vi "Insert Into Subpanel.vi"(8 "error in (no error)":errorcluster, 9 "Insertion Request Time":timestamp, 10 "Viewable":refnum<class "IViewable.lvclass">, 11 "Protected Subpanel":T1) -> (0 "error out":errorcluster, 1 "Inserted?":bool, 2 "Viewable Out":refnum<class "IViewable.lvclass">, 3 "Protected Subpanel":T1)   [LabVIEW 2020, in "MVA Framework.lvlib" / "IViewable.lvlib" / "ProtectedSubpanel.lvclass"]
doc: "插入子面板"
uses:
  ProtectedSubpanel.lvclass
  Protected Subpanel Reference.ctl
  IViewable/IViewable.lvclass
  IViewable/IViewable.lvclass/IViewable.ctl
  ProtectedSubpanel.lvclass/ProtectedSubpanel.ctl
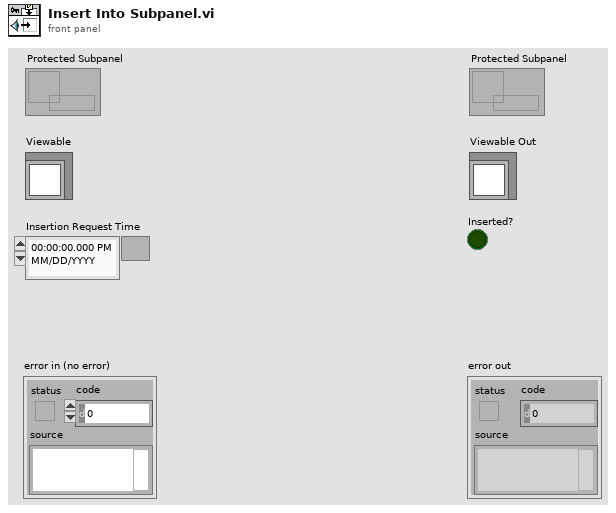
[diagram p1: front panel]
types:
  T1 = typedef "MVA Framework.lvlib/IViewable.lvlib/ProtectedSubpanel.lvclass/Protected Subpanel Reference.ctl" = refnum<data-value>
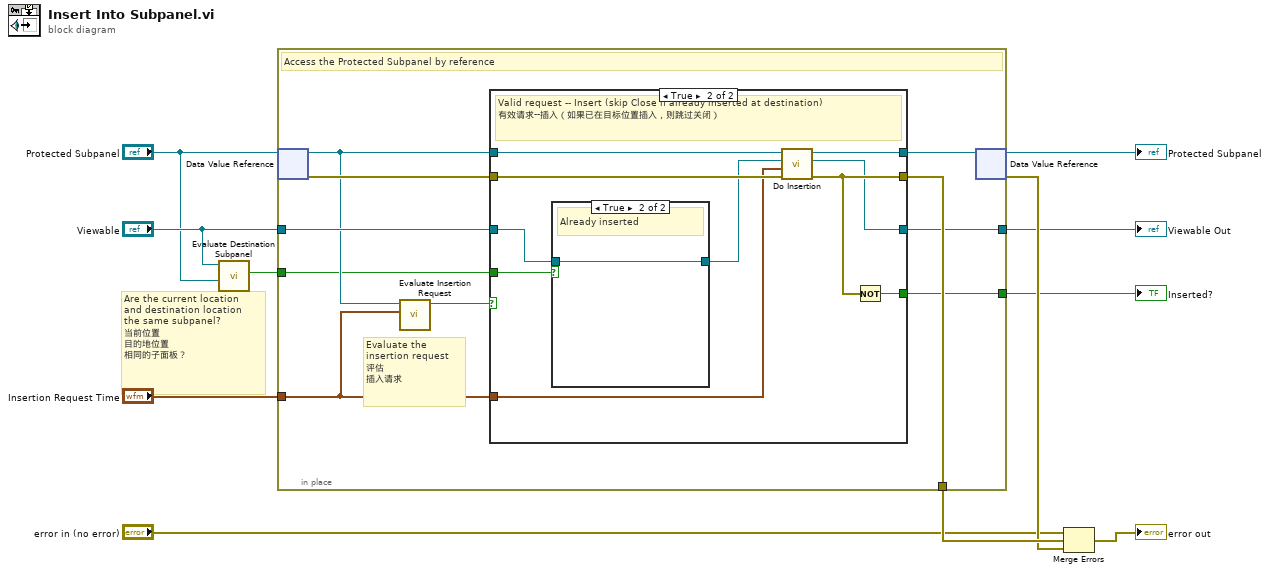
[diagram p0: block diagram]
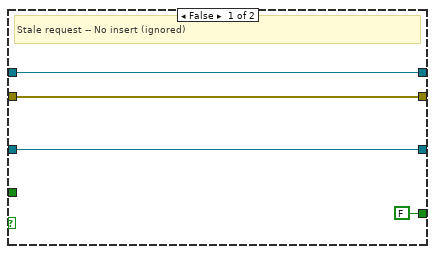
[diagram p2: hidden frame]
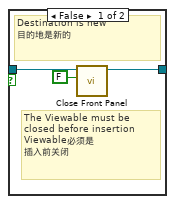
[diagram p3: hidden frame]
diagram:
  # "Are the current location\nand destination location\nthe same subpanel?\n当前位置\n目的地位置\n相同的子面板？"
  n1 = call "Evaluate Destination Subpanel.vi"("Destination Subpanel"="Protected Subpanel", "Viewable in"="Viewable") -> ("Already Inserted?"=w2:bool)  [unwired: 9 in]
  n2 = in-place {
    in-place-border: "Viewable" -> [w15]
    in-place-border: "Insertion Request Time" -> [w17]
    in-place-border: [w18] -> w8
    in-place-border: [w16] -> w6
    in-place-border: [w13] -> w5
    in-place-border: w2 -> [w12]
    # "Evaluate the\ninsertion request\n评估\n插入请求"
    # "Access the Protected Subpanel by reference"
    n3 = in-place-dvr #1("Protected Subpanel") -> (w14:refnum<class "ProtectedSubpanel.lvclass">, w19:errorcluster)
    n4 = call "Evaluate Insertion Request.vi"("Insertion Request Time"=w17, "ProtectedSubpanel"=w14) -> ("Perform Insertion?"=w20:bool)  [unwired: 9 in]
    n5 = case shown="True" w20 {
      tunnel: [w25 w35] -> w21
      tunnel: w14 -> [w25 w34]
      tunnel: w19 -> [w24 w33]
      tunnel: [w24 w32] -> w18
      tunnel: w17 -> [_ w30]
      tunnel: [FALSE w31] -> w16
      tunnel: w15 -> [w22 w28]
      tunnel: [w22 w29] -> w13
      tunnel: w12 -> [_ w26]
      frame False {
        # "Stale request -- No insert (ignored)"
      }
      frame True {
        # "Valid request -- Insert (skip Close if already inserted at destination)\n有效请求--插入（如果已在目标位置插入，则跳过关闭）"
        n6 = case shown="True" w26 {
          tunnel: w28 -> [w37 w39]
          tunnel: [w36 w39] -> w27
          frame False {
            # "The Viewable must be\nclosed before insertion\nViewable必须是\n插入前关闭"
            # "Destination is new\n目的地是新的"
            n7 = call-dynamic "Close Front Panel.vi"("Hide? (F)"=FALSE, "IViewable in"=w37) -> ("IViewable out"=w36:refnum<class "IViewable.lvclass">)  [unwired: 8 in, 1 out]
          }
          frame True {
            # "Already inserted"
          }
        }
        n8 = call "Do Insertion.vi"("error in (no error)"=w33, "Insertion Request Time"=w30, "Viewable"=w27, "ProtectedSubpanel in"=w34) -> ("error out"=w32:errorcluster, "Viewable Out"=w29:refnum<class "IViewable.lvclass">, "ProtectedSubpanel out"=w35:refnum<class "ProtectedSubpanel.lvclass">)  [unwired: 5 in]
        n9 = Not(x=w32) -> (.not. x?=w31:bool)
      }
    }
    n10 = in-place-dvr #1(w21) -> (→"Protected Subpanel":T1, w7:errorcluster)
  }
  "Inserted?" <- w6
  "Viewable Out" <- w5
  n11 = Merge Errors("error in (no error)", w8, w7) -> (→"error out":errorcluster)
